vi "TestNoParameterFunctions.vi"(8 "error in (no error)":errorcluster) -> (0 "error out":errorcluster)   [LabVIEW 2020]
uses:
  <vilib>/addons/_JKI Toolkits/Caraya/classes/Test/Test.lvclass
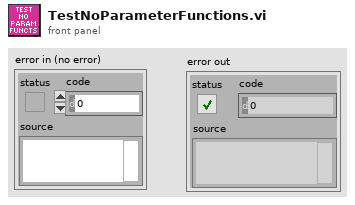
[diagram p1: front panel]
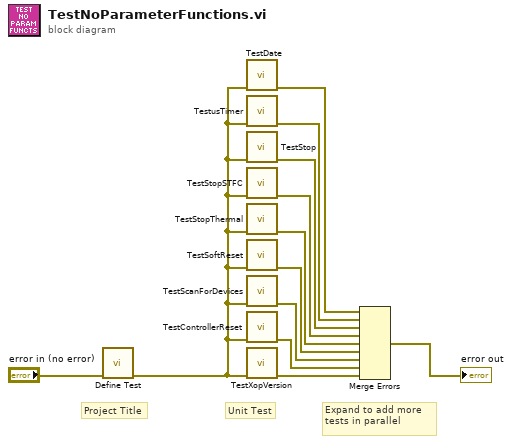
[diagram p0: block diagram]
diagram:
  # "Expand to add more tests in parallel"
  # "Unit Test"
  # "Project Title"
  n1 = call <vilib>:"Define Test.vi"("error in (no error)"="error in (no error)") -> ("error out"=w1:errorcluster)  [unwired: 10 in]
  n2 = call "TestDate.vi"("error in (no error)"=w1) -> ("error out"=w2:errorcluster)  [unwired: 10 in]
  n3 = call "TestusTimer.vi"("error in (no error)"=w1) -> ("error out"=w3:errorcluster)  [unwired: 10 in]
  n4 = call "TestStop.vi"("error in (no error)"=w1) -> ("error out"=w4:errorcluster)  [unwired: 10 in]
  n5 = call "TestStopSTFC.vi"("error in (no error)"=w1) -> ("error out"=w5:errorcluster)  [unwired: 10 in]
  n6 = call "TestStopThermal.vi"("error in (no error)"=w1) -> ("error out"=w6:errorcluster)  [unwired: 10 in]
  n7 = call "TestSoftReset.vi"("error in (no error)"=w1) -> ("error out"=w7:errorcluster)  [unwired: 10 in]
  n8 = call "TestScanForDevices.vi"("error in (no error)"=w1) -> ("error out"=w8:errorcluster)  [unwired: 10 in]
  n9 = call "TestControllerReset.vi"("error in (no error)"=w1) -> ("error out"=w9:errorcluster)  [unwired: 10 in]
  n10 = call "TestXopVersion.vi"("error in (no error)"=w1) -> ("error out"=w10:errorcluster)  [unwired: 10 in]
  n11 = Merge Errors(w2, w3, w4, w5, w6, w7, w8, w9, w10) -> (→"error out":errorcluster)
